vi "Poziomy.vi"(1 "Miny":i32=8, 2 "cons":i32=12, 3 "Mina nr1":i32=9, 4 "Rozmiar":i32=6) -> (0 "Array":i32[][](array[numeric]))   [LabVIEW 2021]
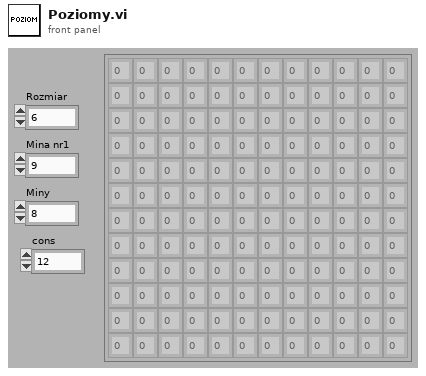
[diagram p1: front panel]
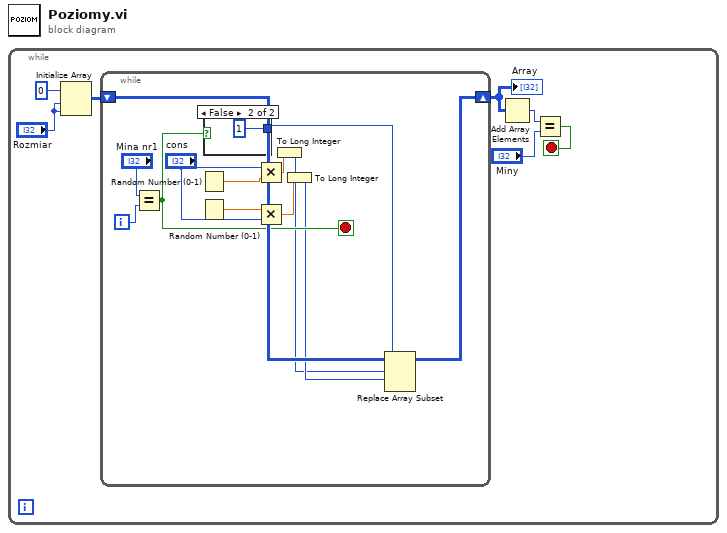
[diagram p0: block diagram]
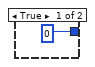
[diagram p2: hidden frame]
diagram:
  n1 = while {
    stop <- w4 stop-if-true
    n2 = Initialize Array(0, "Rozmiar", "Rozmiar") -> (w6:i32[][])
    n3 = while {
      shift-right: [w19] -> w1
      shift-left: w6 -> [w18]
      i -> [w16]
      stop <- w15 stop-if-true
      n4 = Equal?(x="Mina nr1", y=w16) -> (x = y?=w15:bool)
      n5 = Random Number (0-1)() -> (number: 0 to 1=w11:dbl)
      n6 = Random Number (0-1)() -> (number: 0 to 1=w10:dbl)
      n7 = case shown="False" w15 {
        tunnel: [0 1] -> w20
        frame True {
        }
        frame False {
        }
      }
      n8 = Multiply(x="cons", y=w11) -> (x*y=w12:dbl)
      n9 = Multiply(x=w10, y="cons") -> (x*y=w13:dbl)
      n10 = To Long Integer(number=w12) -> (32bit integer=w8:i32)
      n11 = To Long Integer(number=w13) -> (32bit integer=w9:i32)
      n12 = Replace Array Subset(array=w18, new element=w20, index (row)=w8, index (col)=w9) -> (w19:i32[][])
    }
    "Array" <- w1
    n13 = Add Array Elements(numeric array=w1) -> (sum=w2:i32)
    n14 = Equal?(x=w2, y="Miny") -> (x = y?=w4:bool)
  }
